vi "ConvertSensitivityToString.vi"(1 "Sensitivity":dbl) -> (0 "Sensitivity String":string)   [LabVIEW 2016, in "SR7270 Drivers.lvlib" / "SR7270 Drivers.lvclass"]
uses:
  SR7270 Drivers.lvclass
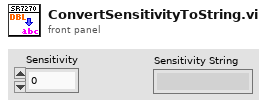
[diagram p1: front panel]
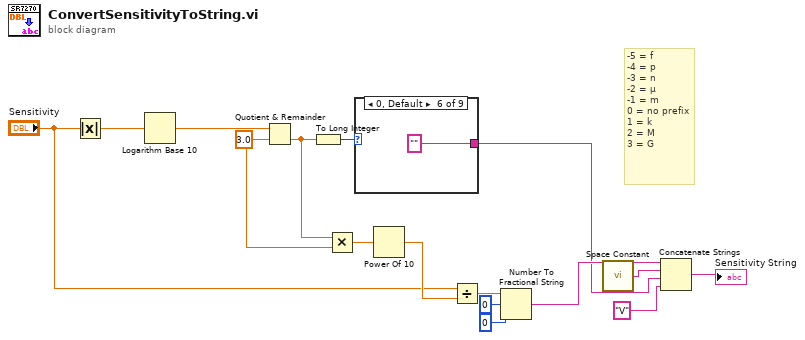
[diagram p0: block diagram]
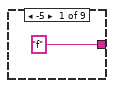
[diagram p2: hidden frame]
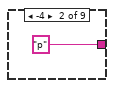
[diagram p3: hidden frame]
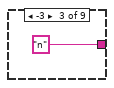
[diagram p4: hidden frame]
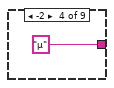
[diagram p5: hidden frame]
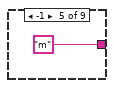
[diagram p6: hidden frame]
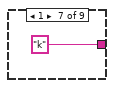
[diagram p7: hidden frame]
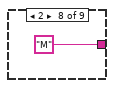
[diagram p8: hidden frame]
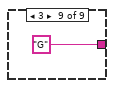
[diagram p9: hidden frame]
diagram:
  w13 = 3.0 ("y")
  # "-5 = f\n-4 = p\n-3 = n\n-2 = µ\n-1 = m\n0 = no prefix\n1 = k\n2 = M\n3 = G"
  n1 = Absolute Value(x="Sensitivity") -> (abs(x)=w10:dbl)
  n2 = Logarithm Base 10(1:w10) -> (0:w16:dbl)
  n3 = Quotient & Remainder(x=w16, y=w13) -> (floor(x/y)=w12:dbl)  [unwired: 1 out]
  n4 = To Long Integer(number=w12) -> (32bit integer=w15:i32)
  n5 = Multiply(x=w12, y=w13) -> (x*y=w14:dbl)
  n6 = case shown="0, Default" w15 {
    tunnel: ["f" "p" "n" "µ" "m" "" "k" "M" "G"] -> w4
    frame -5 {
    }
    frame -4 {
    }
    frame -3 {
    }
    frame -2 {
    }
    frame -1 {
    }
    frame 0, Default {
    }
    frame 1 {
    }
    frame 2 {
    }
    frame 3 {
    }
  }
  n7 = Power Of 10(x=w14) -> (10^x=w11:dbl)
  n8 = Divide(x="Sensitivity", y=w11) -> (x/y=w8:dbl)
  n9 = Number To Fractional String(number=w8, width (-)=i16 0, precision (6)=i16 0) -> (F-format string=w7:string)  [unwired: 1 in]
  n10 = call <vilib>:"Space Constant.vi"() -> ("String"=w6:string)
  n11 = Concatenate Strings(w7, w6, w4, "V" ("string")) -> (→"Sensitivity String":string)
